vi "Scripting_RelinkSubVI.vi"(10 "error in":errorcluster, 11 "SubVIIn":refnum<vi>) -> (2 "error out":errorcluster, 3 "SubVIOut":refnum<vi>)   [LabVIEW 2020]
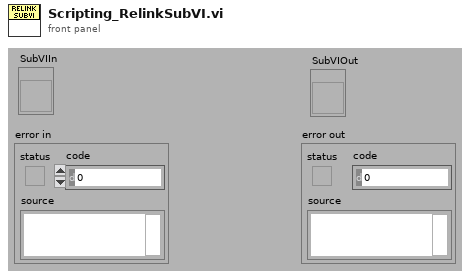
[diagram p1: front panel]
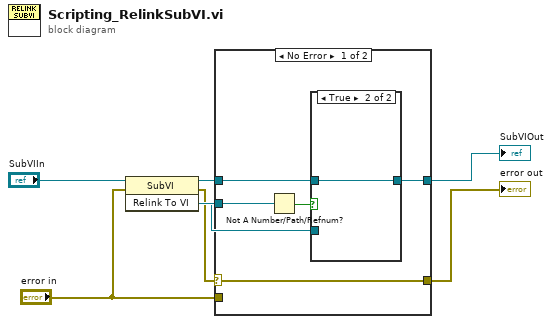
[diagram p0: block diagram]
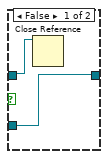
[diagram p2: hidden frame]
diagram:
  n1 = invoke class="SubVI" method="Relink To VI"(reference="SubVIIn", error in="error in") -> (reference out=w5:refnum<vi>, error out=w3:errorcluster, "Relink To VI"=w7:refnum<vi>)  [unwired: 1 in]
  n2 = case shown="No Error" w3 {
    selector: w3 -> [w8 _]
    tunnel: w7 -> [w12 _]
    tunnel: [w11 w16] -> w6
    tunnel: w5 -> [w10 w16]
    tunnel: [w8 w17] -> w2
    tunnel: "error in" -> [_ w17]
    frame No Error {
      n3 = Not A Number/Path/Refnum?(number/path/refnum=w12) -> (NaN/Path/Refnum?=w9:bool)
      n4 = case shown="True" w9 {
        tunnel: w10 -> [w13 w15]
        tunnel: [w14 w15] -> w11
        tunnel: w12 -> [w14 _]
        frame False {
          n5 = Close Reference(reference=w13) -> ()  [unwired: 1 in, 1 out]
        }
        frame True {
        }
      }
    }
    frame Error {
    }
  }
  "error out" <- w2
  "SubVIOut" <- w6
